vi "Write @Energy.vi"(8 "error in (no error)":errorcluster, 10 "@Energy":dbl[unit]=10.0 format="%#_13g", 11 "HIJ Vision Fluence Cam in":refnum<class "HIJ Vision Fluence Cam.lvclass">) -> (0 "error out":errorcluster, 3 "HIJ Vision Fluence Cam out":refnum<class "HIJ Vision Fluence Cam.lvclass">)   [LabVIEW 2014, in "HIJ Vision Fluence Cam.lvlib" / "HIJ Vision Fluence Cam.lvclass"]
uses:
  HIJ Vision Fluence Cam.lvclass
  HIJ Vision Fluence Cam.lvclass/HIJ Vision Fluence Cam.ctl
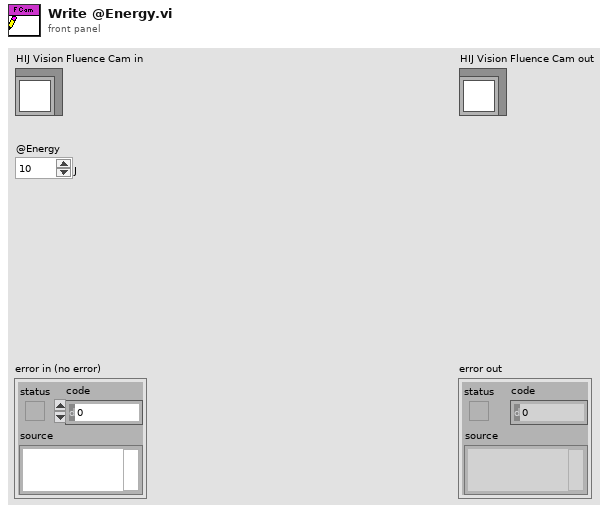
[diagram p1: front panel]
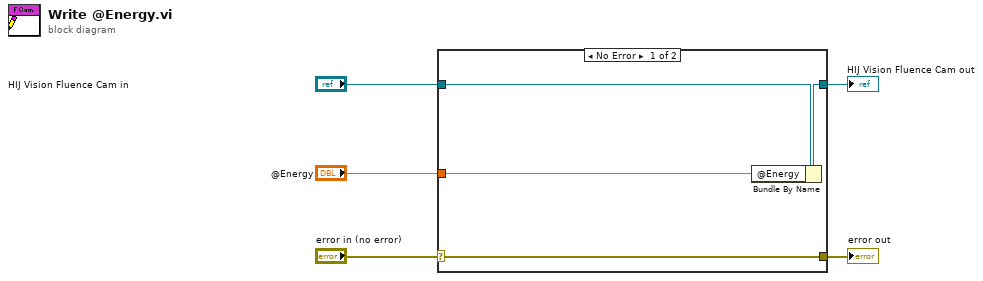
[diagram p0: block diagram]
diagram:
  n1 = case shown="No Error" "error in (no error)" {
    selector: "error in (no error)" -> [w9 w10]
    tunnel: [w9 w10] -> w4
    tunnel: [w7 w11] -> w2
    tunnel: "HIJ Vision Fluence Cam in" -> [w8 w11]
    tunnel: "@Energy" -> [w6 _]
    frame No Error {
      n2 = Bundle By Name(cluster=w8, "@Energy"=w6) -> (w7:refnum<class "HIJ Vision Fluence Cam.lvclass">)
    }
    frame Error {
    }
  }
  "error out" <- w4
  "HIJ Vision Fluence Cam out" <- w2
